vi "FPGA_LUT_Test1.vi"() -> ()   [LabVIEW 2014]
uses:
  <vilib>/Platform/TimedLoop/XDataNode/timing_clust.ctl
  <vilib>/Platform/TimedLoop/XDataNode/nitl_modes.ctl
  <vilib>/Platform/TimedLoop/XDataNode/wakeup.ctl
  <vilib>/rvi/DataTransferAndStorage/Container/Common/niFpgaContainerGetUniqueNameForEmu.vi
  <vilib>/rvi/DataTransferAndStorage/Container/Common/niFpgaContainerSetEmuInfo.vi
  <vilib>/rvi/eio/common/nirviEmuReportErrorAndStop.vi
  <vilib>/rvi/Emulation/niFpgaSctlEmulationGetInTimedLoop.vi
  <vilib>/rvi/Emulation/niFpgaEmulationReportErrorSimple.vi
  <vilib>/rvi/Emulation/niFpgaGetClockAttributes.vi
  <vilib>/rvi/Emulation/niFpgaCriticalErrorInLSC.vi
  <vilib>/rvi/DataTransferAndStorage/Container/Common/niFpgaContainerExecOnDevCompGetState.vi
  <vilib>/rvi/Emulation/niFpgaEmulationIsFPGAContextNoSignature.vi
  <vilib>/rvi/Emulation/niFpgaProcessEmulError.vi
  <vilib>/rvi/errors/nirviReportUnexpectedCaseInternalError (U32).vi
  <vilib>/rvi/Memory/Memory_Emulation/niFpgaMemoryEmulationCacheClearOnFirstRun.vi
  <vilib>/rvi/Memory/Memory_Emulation/nirvimemoryEmulationManagerCache_MakeExclusive.vi
  <vilib>/rvi/Memory/Memory_Emulation/niFpgaMemoryEmulationValidateCache.vi
  <vilib>/rvi/Memory/Memory_Emulation/nirvimemoryEmulationManagerCache_InsertValue.vi
  <vilib>/Utility/error.llb/Clear Errors.vi
  <vilib>/rvi/Memory/Memory_Emulation/nirvimemoryEmulationManagerCache_ReleaseExclusive.vi
  <vilib>/rvi/Memory/Memory_Emulation/nirvimemoryEmulationManagerCache_GetValue.vi
  <vilib>/rvi/Memory/Memory_Emulation/nirvimemoryEmulationManagerCache_SetValue.vi
  <vilib>/rvi/Emulation/niFpgaSctlEmulationResourceMgr.vi
  <vilib>/Platform/TimedLoop/XDataNode/XDataNode.xnode
  <vilib>/rvi/LocalResourceManager/LocalResourceManager.xnode
  <vilib>/rvi/DataTransferAndStorage/Container/XNode/niFpgaContainer.xnode
  <vilib>/rvi/Memory/Memory_Emulation/niFpgaMemoryEmulationRefIn.vi
  <vilib>/Platform/TimedLoop/XDataNode/XDNodeRunTimeDep.lvlib
panel:
  out "Array":i16[](array[numeric])
  out "TimeDelta":u32
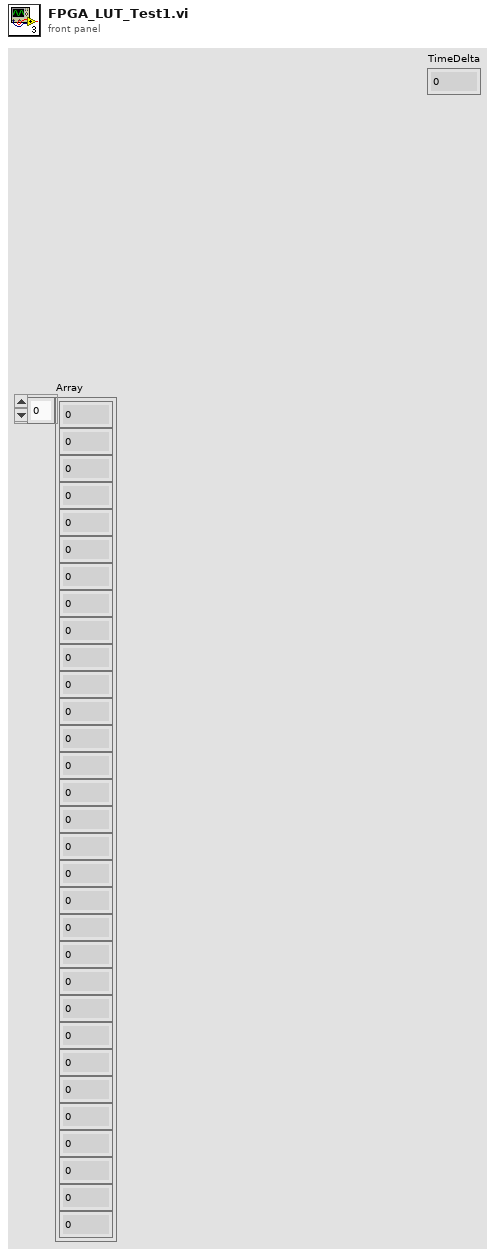
[diagram p1: front panel]
types:
  T1 = typedef "XDNodeRunTimeDep.lvlib/timing_clust.ctl" = cluster{"Expected End [f-1]":u64, "Actual End [f-1]":u64, "Finished Late? [f-1]":bool, "Expected End [i-1]":u64, "Actual End [i-1]":u64, "Finished Late? [i-1]":bool, "Expected Start [i]":u64, "Actual Start [i]":u64, "Expected Start [f]":u64, "Actual Start [f]":u64, "Source Name":string, "Structure Name":string, "Period":i64, "Deadline":i64, "Offset":i64, "Start":i64, "Priority":i32, "Timeout":i32, "Mode":T2, "Wakeup Reason":T3, "Error":errorcluster, "Source Type":string, "Secondary Source Type":string, "Global End Time":u64, "Global Start Time":u64, "Frame Duration":u64, "Iteration Duration":u64, "Assigned CPU":i32, "I/O Scan Engine Mode":u32}
  T2 = typedef "XDNodeRunTimeDep.lvlib/nitl_modes.ctl" = enum32{"No Change", "Process missed periods, maintain original phase", "Discard missed periods, maintain original phase", "Process missed periods, ignore original phase", "Discard missed periods, ignore original phase"}
  T3 = typedef "XDNodeRunTimeDep.lvlib/wakeup.ctl" = enum32{"Normal", "Aborted", "Asynchronous wakeup", "Timing source error", "Timed loop error", "Timeout"}
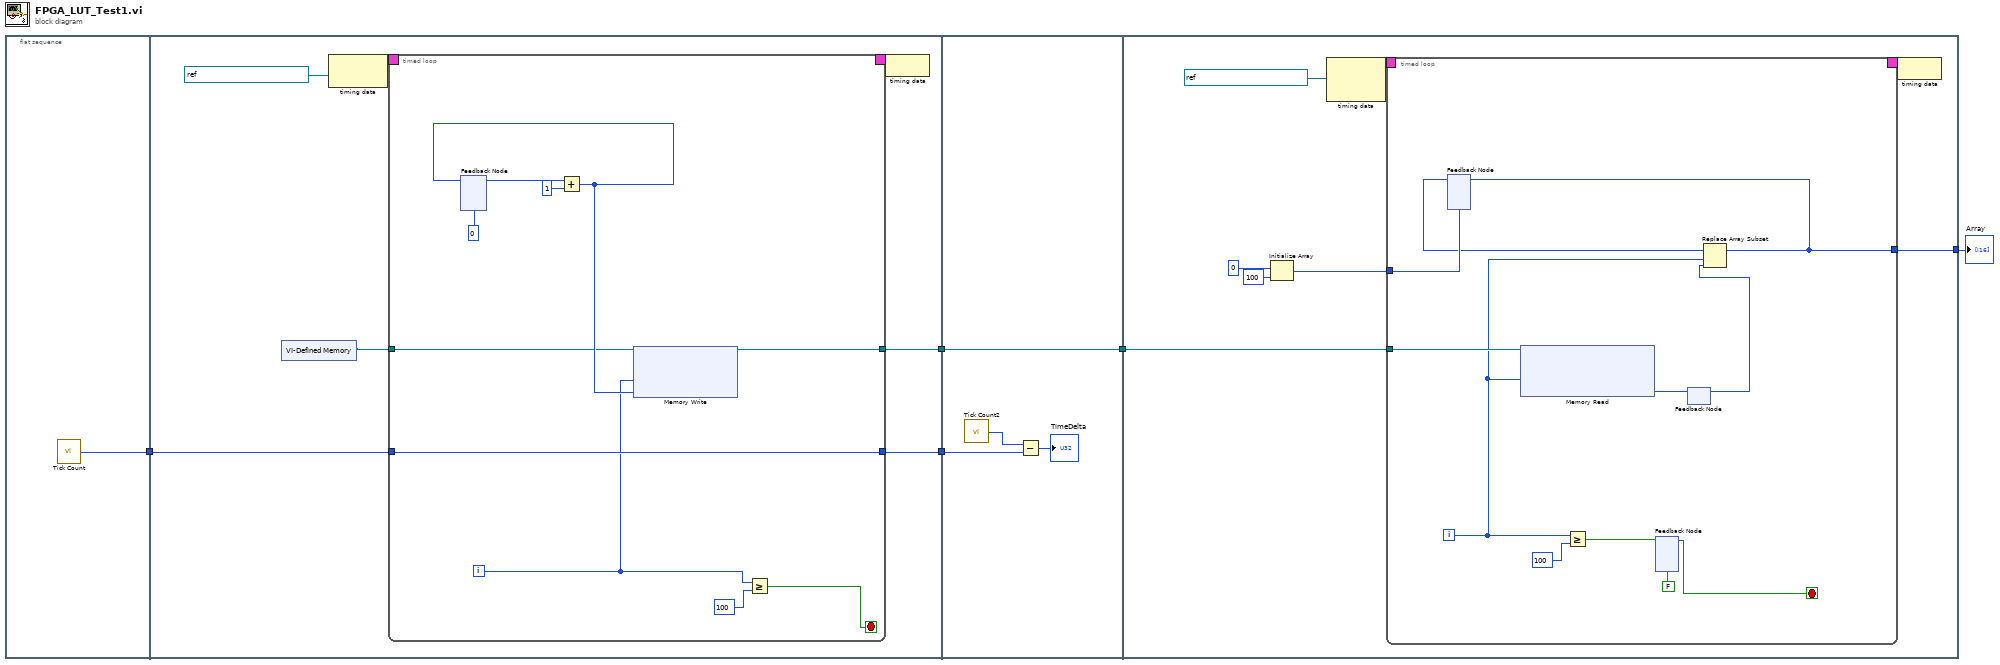
[diagram p0: block diagram]
diagram:
  n1 = flat-sequence {
    tunnel: [w6] -> w5
    tunnel: w5 -> [w10]
    tunnel: [w9] -> w4
    tunnel: [w7] -> w3
    tunnel: w4 -> [w33]
    tunnel: w3 -> [w30]
    tunnel: [w30] -> w2
    tunnel: w2 -> [w38]
    tunnel: [w34] -> w1
    frame #0 {
      n2 = call "Tick Count"() -> ("Tick Count(uSec)"=w6:u32)
    }
    frame #1 {
      n3 = xnode "VI-Defined Memory"() -> ("Memory Out"=w8:refnum<k21>)
      n4 = node-c288(refnum<k21> "40 MHz Onboard Clock" ("Source Name")) -> (w13:T1)
      n5 = timed-loop {
        timing: w13 -> [_]
        timing-out: [_] -> w12
        tunnel: w10 -> [w18]
        tunnel: [w18] -> w9
        tunnel: w8 -> [w16]
        tunnel: [w14] -> w7
        i -> [w15]
        stop <- w19 stop-if-true
        n6 = feedback #1(i16 0) -> (w22:i16)
        n7 = Add(x=w22, y=i16 1) -> (x+y=w17:i16)
        n8 = feedback-in #1(w17) -> ()
        n9 = xnode ("Memory Write")("Address"=w15, "Data"=w17, "Memory In"=w16) -> ("Memory Out"=w14:refnum<k21>)
        n10 = Greater Or Equal?(x=w15, y=100) -> (x >= y?=w19:bool)
      }
      n11 = node-c288(w12) -> ()
    }
    frame #2 {
      n12 = call "Tick Count2"() -> ("Tick Count(uSec)"=w32:u32)
      n13 = Subtract(x=w32, y=w33) -> (x-y=→"TimeDelta":u32)
    }
    frame #3 {
      n14 = Initialize Array(i16 0, 100 ("dimension size")) -> (w35:i16[])
      n15 = node-c288(refnum<k21> "40 MHz Onboard Clock" ("Source Name")) -> (w41:T1)  [unwired: 1 in]
      n16 = timed-loop {
        timing: w41 -> [_]
        timing-out: [_] -> w40
        tunnel: w38 -> [w52]
        tunnel: w35 -> [w45]
        tunnel: [w46] -> w34
        i -> [w47]
        stop <- w48 stop-if-true
        n17 = feedback #2(w45) -> (w44:i16[])
        n18 = xnode ("Memory Read")("Address"=w47, "Memory In"=w52) -> ("Data"=w43:i16)  [unwired: 1 out]
        n19 = Greater Or Equal?(x=w47, y=100) -> (x >= y?=w50:bool)
        n20 = feedback #3(FALSE) -> (w48:bool)
        n21 = feedback-in #3(w50) -> ()
        n22 = feedback-in #4(w43) -> ()
        n23 = feedback #4() -> (w42:i16)  [unwired: 1 in]
        n24 = Replace Array Subset(array=w44, new element=w42, index=w47) -> (w46:i16[])
        n25 = feedback-in #2(w46) -> ()
      }
      n26 = node-c288(w40) -> ()
    }
  }
  "Array" <- w1
